vi "JV PJVS GUI control.vi"() -> ()   [LabVIEW 2020]
uses:
  DataSocketCluster external.ctl
  <instrlib>/niFgen/niFgen.llb/niFgen_ctl Sample Clock Source Values (Ring).ctl
panel:
  out "actual FGEN handle":refnum<k15> caption="Instrument Handle Out"
  in  "?":T1(tab)
  in  "Set AC wave":bool
  in  "Steps on PJVS curve":u32=100
  in  "Frequency (Hz)":dbl=100.0 format="%#_10g"
  in  "Send AC":bool
  in  "Send DC string":bool
  in  "DC-String":string="SETDC_MMMMMMMMMMOO"
  in  "Send 0 V to bias source":bool
  in  "Amplitude (V)":dbl=1.0
  in  "Stop trigger":bool caption="Stop"
  in  "Amplitude":dbl=2.0 format="%0_3g"
  in  "Frequency":dbl=1000000.0 format="%.2p"
  in  "Standard Waveform":u16(ring) items=["Sine", "Square", "Triangle", "Ramp Up", "Ramp Down", "DC", "Noise"]
  in  "FGEN Resource Name":refnum<k15>
  in  "Start trigger":bool
  in  "Channel":string="0"
  in  "Source (Onboard Clock)":T2="OnboardClock"
  in  "This machine (client)":string="localhost"
  in  "Name of computer":string="CZC105BD8M"
  in  "TimeOut Time (s)":dbl=30.0 format="%.2f"
  out "Response from NPL bias source":string
  out "error out":errorcluster {"code" format="%.0x"}
  out "machine":T3 {"TimeStamp" format="%.2f"}
  out "Voltage at each step on PJVS curve":dbl[](array[numeric]) format="%#_16g"
  out "Return time interval on PJVS step":string
  out "Calculated time on PJVS step (smallest value is 17)":u32=100
  in  "Quit":bool
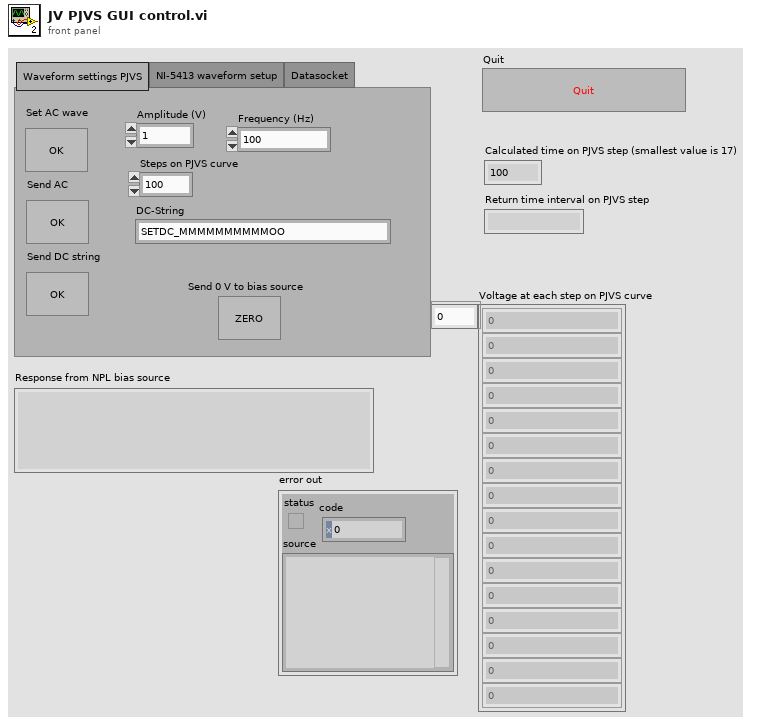
[diagram p1: front panel]
types:
  T1 = enum32{"Waveform settings PJVS", "NI-5413 waveform setup", "Datasocket"}
  T2 = typedef "niFgen_ctl Sample Clock Source Values (Ring).ctl" = string
  T3 = typedef "DataSocketCluster external.ctl" = cluster{"Server Machine":string, "Client Machine":string, "Data":string, "TimeStamp":dbl, "Count":i32, "Target Process":string}
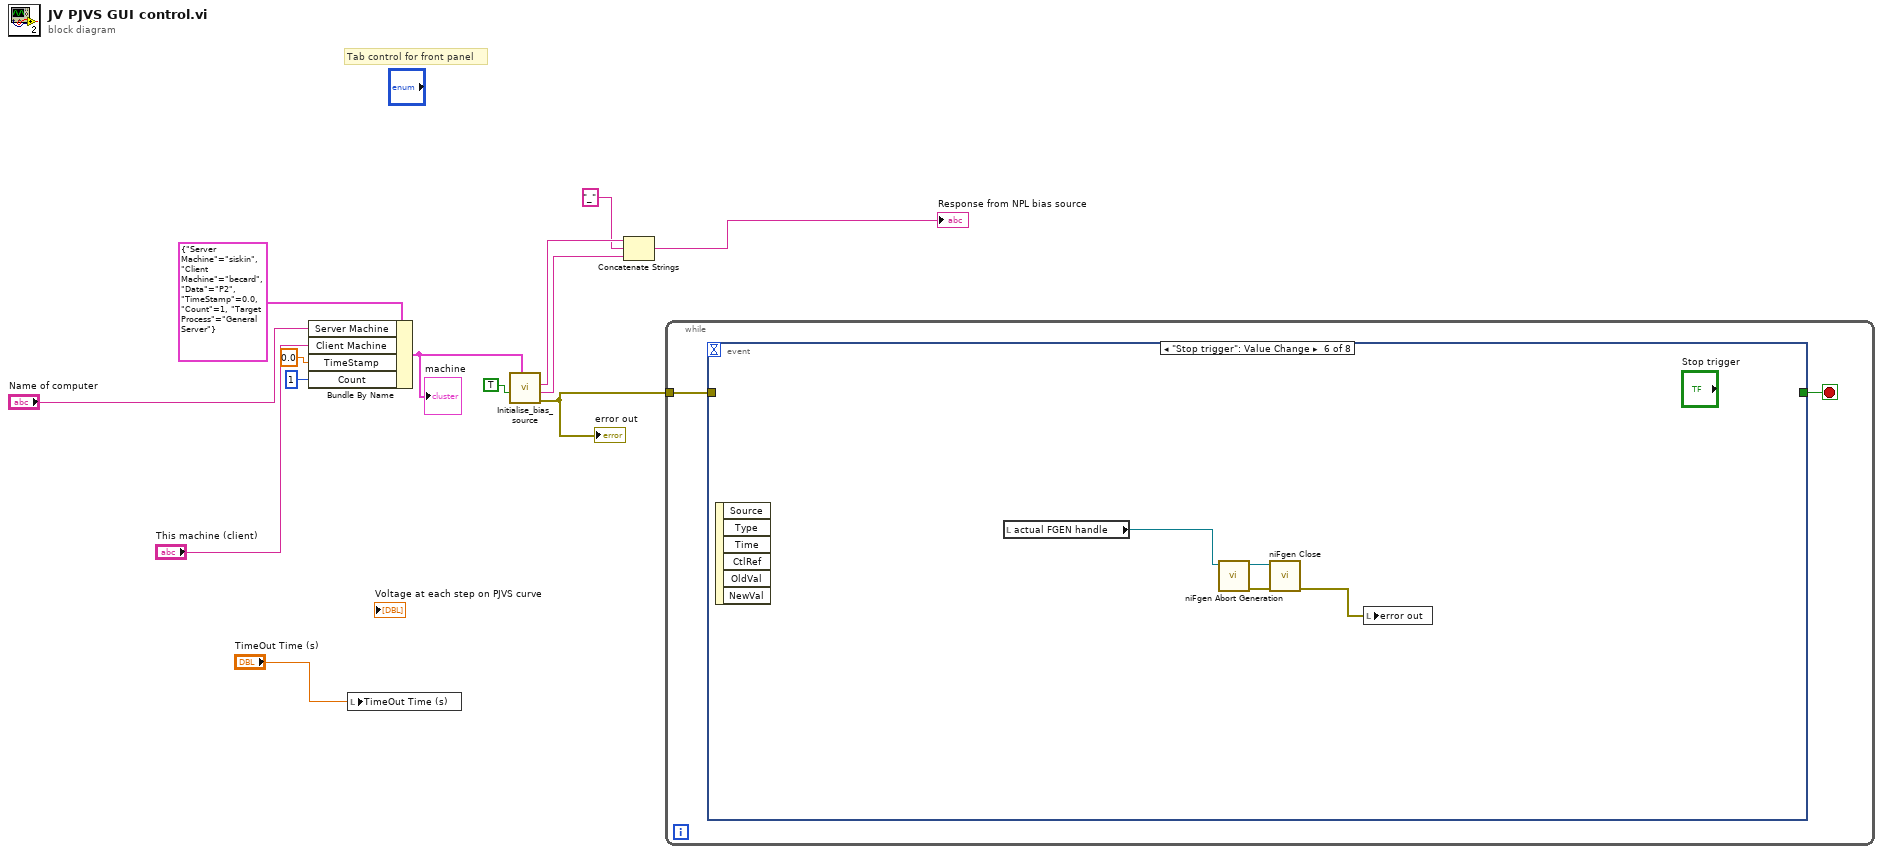
[diagram p0: block diagram]
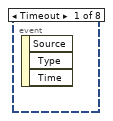
[diagram p2: hidden frame]
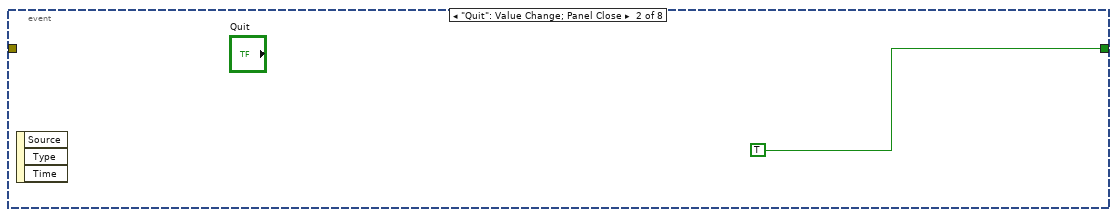
[diagram p3: hidden frame]
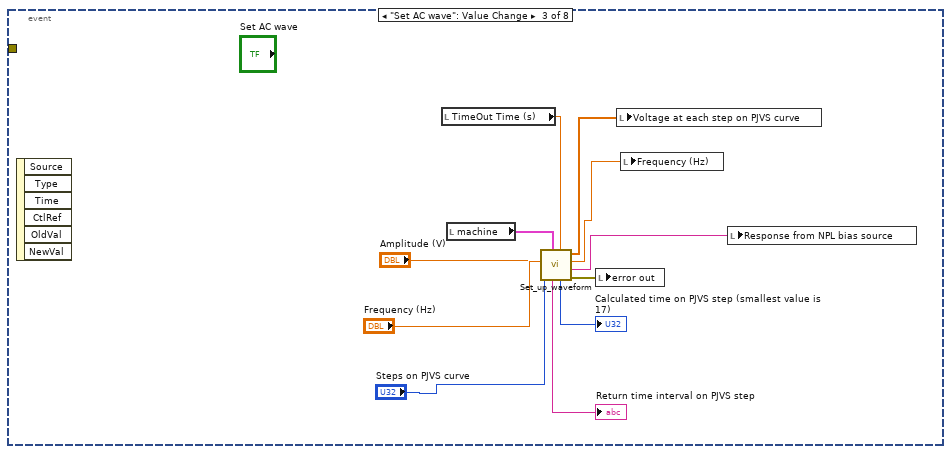
[diagram p4: hidden frame]
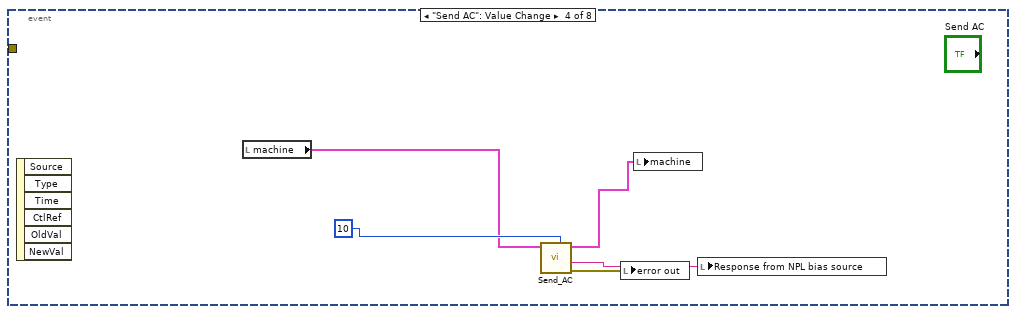
[diagram p5: hidden frame]
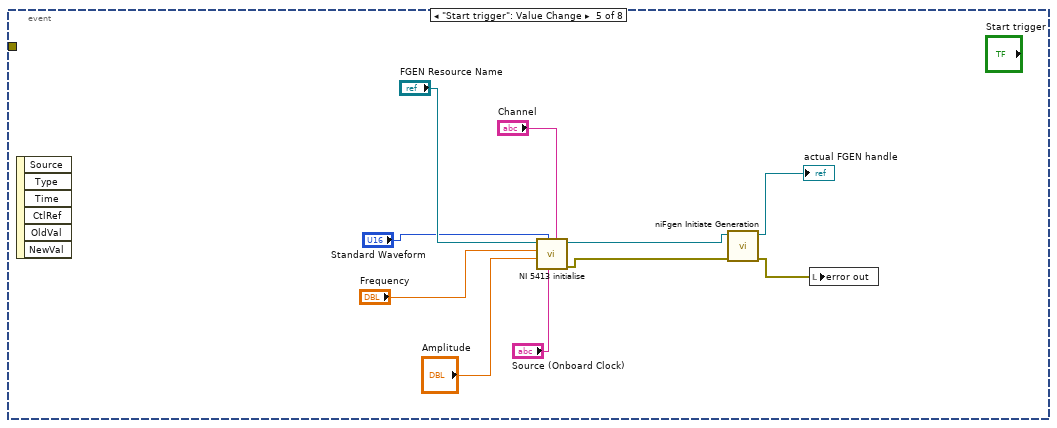
[diagram p6: hidden frame]
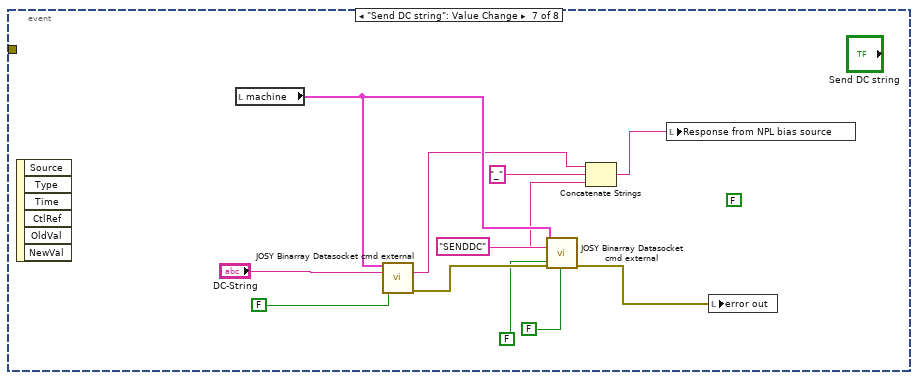
[diagram p7: hidden frame]
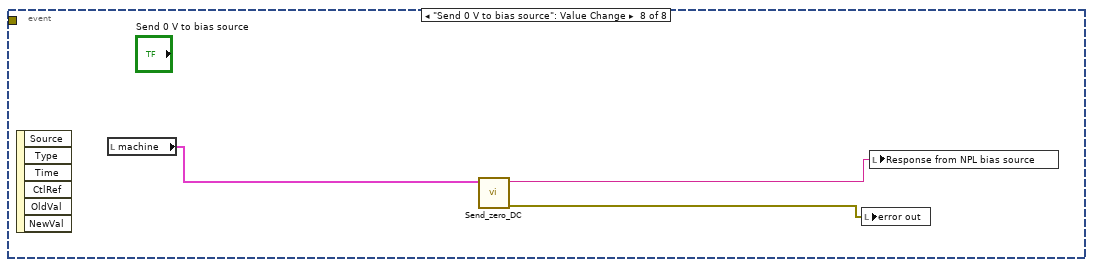
[diagram p8: hidden frame]
diagram:
  # "Tab control for front panel"
  n1 = Bundle By Name(cluster=T3 {"Server Machine"="siskin", "Client Machine"="becard", "Data"="P2", "TimeStamp"=0.0, "Count"=1, "Target Process"="General Server"} ("DataSocketCluster In"), "Server Machine"="Name of computer", "Client Machine"="This machine (client)", "TimeStamp"=0.0, "Count"=1) -> (w8:T3)
  "machine" <- w8
  n2 = local write "TimeOut Time (s)"("TimeOut Time (s)") -> ()
  n3 = call "Initialise_bias_source.vi"("output cluster"=w8, "Load bias parameters"=TRUE) -> ("error out"=w7:errorcluster, "Response to Load bias parameters"=w5:string, "Response Initialise"=w3:string)  [unwired: 7 in]
  "error out" <- w7
  n4 = Concatenate Strings(w3, "_" ("string"), w5) -> (→"Response from NPL bias source":string)
  n5 = while {
    tunnel: w7 -> [w14]
    stop <- w15 stop-if-true
    n6 = event shown="[5] \"Stop trigger\": Value Change" {
      selector: _ -> [_ _ _ _ _ _ _ _]
      dyn-events: _ -> [_ _ _ _ _ _ _ _]
      timeout: _ -> [_ _ _ _ _ _ _ _]
      tunnel: [_ TRUE _ _ _ _ _ _] -> w15
      tunnel: w14 -> [_ _ _ _ _ _ _ _]
      event Timeout {
        n7 = event-data() -> ()  [unwired: 1 in, 3 out]
      }
      event "Quit": Value Change; Panel Close {
        n8 = event-data() -> ()  [unwired: 1 in, 3 out]
      }
      event "Set AC wave": Value Change {
        n9 = event-data() -> ()  [unwired: 1 in, 6 out]
        n10 = local read "TimeOut Time (s)"() -> (w25:dbl)
        n11 = local read "machine"() -> (w21:T3)
        n12 = call "Set_up_waveform.vi"("TimeOut Time (s)"=w25, "DataSocketCluster In"=w21, "Steps on PJVS curve"="Steps on PJVS curve", "Frequency (Hz)"="Frequency (Hz)", "Amplitude (V)"="Amplitude (V)") -> ("error IO"=w22:errorcluster, "Returned number of steps on PJVS curve"=w23:string, "Set frequency (Hz)"=w26:dbl, "Voltage at each step on PJVS curve"=w24:dbl[], "Calculated time on step (smallest value is 17)"=→"Calculated time on PJVS step (smallest value is 17)":u32, "Returned time interval on each step"=→"Return time interval on PJVS step":string)  [unwired: 1 in]
        n13 = local write "error out"(w22) -> ()
        n14 = local write "Voltage at each step on PJVS curve"(w24) -> ()
        n15 = local write "Frequency (Hz)"(w26) -> ()
        n16 = local write "Response from NPL bias source"(w23) -> ()
      }
      event "Send AC": Value Change {
        n17 = event-data() -> ()  [unwired: 1 in, 6 out]
        n18 = local read "machine"() -> (w29:T3)
        n19 = call "Send_AC.vi"("milliseconds to wait"=u32 10, "DataSocketCluster In"=w29) -> ("error out"=w31:errorcluster, "Response to SEND AC"=w30:string, "DataSocketCluster out"=w28:T3)  [unwired: 7 in]
        n20 = local write "error out"(w31) -> ()
        n21 = local write "machine"(w28) -> ()
        n22 = local write "Response from NPL bias source"(w30) -> ()
      }
      event "Start trigger": Value Change {
        n23 = event-data() -> ()  [unwired: 1 in, 6 out]
        n24 = call "NI 5413 initialise.vi"("Channel"="Channel", "Source (Onboard Clock)"="Source (Onboard Clock)", "Standard Waveform"="Standard Waveform", "Amplitude"="Amplitude", "Frequency"="Frequency", "FGEN Resource Name"="FGEN Resource Name") -> ("error out"=w36:errorcluster, "Instrument Handle Out"=w34:refnum<k15>)  [unwired: 4 in]
        n25 = call <instrlib>:"niFgen Initiate Generation.vi"("error in (no error)"=w36, "Instrument Handle"=w34) -> ("error out"=w35:errorcluster, "Instrument Handle Out"=→"actual FGEN handle":refnum<k15>)  [unwired: 8 in]
        n26 = local write "error out"(w35) -> ()
      }
      event "Stop trigger": Value Change {
        n27 = event-data() -> ()  [unwired: 1 in, 6 out]
        n28 = local read "actual FGEN handle"() -> (w44:refnum<k15>)
        n29 = call <instrlib>:"niFgen Abort Generation.vi"("Instrument Handle"=w44) -> ("error out"=w46:errorcluster, "Instrument Handle Out"=w45:refnum<k15>)  [unwired: 9 in]
        n30 = call <instrlib>:"niFgen Close.vi"("error in (no error)"=w46, "Instrument Handle"=w45) -> ("error out"=w43:errorcluster)  [unwired: 9 in]
        n31 = local write "error out"(w43) -> ()
      }
      event "Send DC string": Value Change {
        (unwired) FALSE ("String")
        n32 = event-data() -> ()  [unwired: 1 in, 6 out]
        n33 = local read "machine"() -> (w55:T3)
        n34 = call "JOSY Binarray Datasocket cmd external.vi"("DataSocketCluster In"=w55, "Command"="DC-String", "Command has variable"=FALSE) -> ("Reply data"=w47:string, "error out"=w56:errorcluster)  [unwired: 9 in, 2 out]
        n35 = call "JOSY Binarray Datasocket cmd external.vi"("DataSocketCluster In"=w55, "Command"="SENDDC", "error in (no error)"=w56, "Command has variable"=FALSE, "String"=FALSE) -> ("Reply data"=w49:string, "error out"=w54:errorcluster)  [unwired: 7 in, 2 out]
        n36 = Concatenate Strings(w47, "_" ("string"), w49) -> (w48:string)
        n37 = local write "Response from NPL bias source"(w48) -> ()
        n38 = local write "error out"(w54) -> ()
      }
      event "Send 0 V to bias source": Value Change {
        n39 = event-data() -> ()  [unwired: 1 in, 6 out]
        n40 = local read "machine"() -> (w61:T3)
        n41 = call "Send_zero_DC.vi"("machine"=w61) -> ("error out"=w59:errorcluster, "String"=w60:string)  [unwired: 9 in]
        n42 = local write "error out"(w59) -> ()
        n43 = local write "Response from NPL bias source"(w60) -> ()
      }
    }
  }
